vi "HISW_destructor.vi"(8 "error in (no error)":errorcluster, 11 "HISW in":refnum<class "HISW.lvclass">) -> (0 "error out":errorcluster, 3 "HISW out":refnum<class "HISW.lvclass">)   [LabVIEW 2020, in "HISW.lvclass"]
doc: "Close the HISW class and close the Gserver application"
uses:
  HISW.lvclass
  D:/Labview/Sgraph/Sgraph/source/AVPP/AVPP.lvclass
  HISW.lvclass/HISW.ctl
  AVPP/AVPP.lvclass
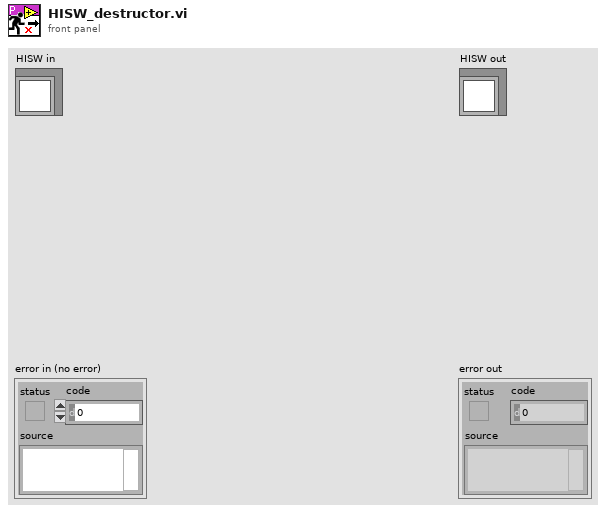
[diagram p1: front panel]
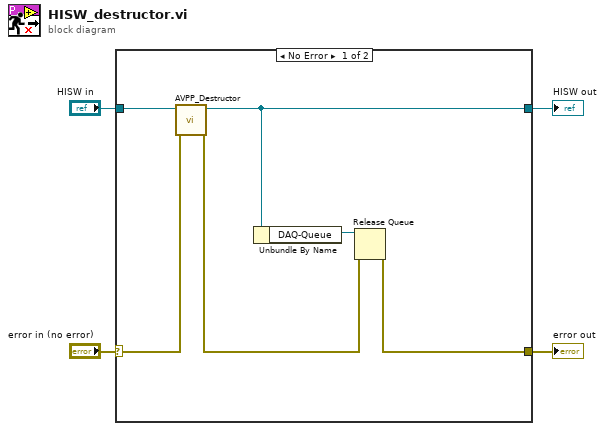
[diagram p0: block diagram]
diagram:
  n1 = case shown="No Error" "error in (no error)" {
    selector: "error in (no error)" -> [w9 w12]
    tunnel: [w5 w12] -> w3
    tunnel: [w8 w11] -> w1
    tunnel: "HISW in" -> [w10 w11]
    frame No Error {
      n2 = call "AVPP_Destructor.vi"("error in (no error)"=w9, "AVPP in"=w10) -> ("error out"=w6:errorcluster, "AVPP out"=w8:refnum<class "HISW.lvclass">)  [unwired: 8 in]
      n3 = Unbundle By Name(w8) -> ("DAQ-Queue"=w7:refnum<queue>)
      n4 = Release Queue(queue=w7, error in (no error)=w6) -> (error out=w5:errorcluster)  [unwired: 1 in, 2 out]
    }
    frame Error {
    }
  }
  "error out" <- w3
  "HISW out" <- w1
